vi "wait autonomous.vi"() -> ()   [LabVIEW 2010, in "Rampage.lvrbt"]
uses:
  Rampage.lvrbt
  <vilib>/NXT/Subs/MotorOutput.ctl
  <vilib>/NXT/NXTIO Xnodes/AddressXNode/NXTIOAddress.xnode
  <vilib>/NXT/Subs/MotorXNode.DC Motor Type.ctl
  <vilib>/NXT/Subs/MotorXNode.2DCMotor.ctl
  <vilib>/NXT/HiTechnic/HiTechnic Controls/HiTechnic Port.ctl
  <vilib>/NXT/Block Support/NXT_InputPort.ctl
  <vilib>/NXT/NXTIO Xnodes/NXTIOXNode/NXTIO.xnode
  <vilib>/NXT/Subs/LVHSConnector.ctl
  <vilib>/NXT/Dual Mode Library/Waits/Wait_Num(msec).vi
  <vilib>/NXT/Dual Mode Library/prims/inRangeAndCoerce/inRangeAndCoerce_int.vi
  <vilib>/NXT/Dual Mode Library/Motors/MotorOn.vi
  <vilib>/NXT/Dual Mode Library/Waits/Wait_Num.vi
  <vilib>/NXT/NXTIO Xnodes/NXTIONodeSubVIs/TETRIX IO Move DC Motors.vi
  <vilib>/NXT/NXTIO Xnodes/NXTIONodeSubVIs/TETRIX IO Stop DC Motors.vi
  <vilib>/NXT/Dual Mode Library/Sensors/Sonar_cm.vi
panel:
  out "Enabled":bool
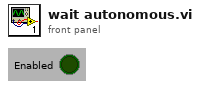
[diagram p1: front panel]
types:
  T1 = typedef "LVHSConnector.ctl" = cluster{"Hardware":string, "Flattened String":string}
  T2 = typedef "MotorOutput.ctl" = u8
  T3 = typedef "MotorXNode.DC Motor Type.ctl" = enum16{"DC Motor"}
  T4 = cluster{"DC Motor":T3, "Address":i16, "Address":i16}
  T5 = typedef "HiTechnic Port.ctl" = cluster{"Port":T6, "MUX Port":u8}
  T6 = typedef "NXT_InputPort.ctl" = u8
  T7 = cluster{"Direction (0-9)":i16, "Signal Strength (Array)":u8[]}
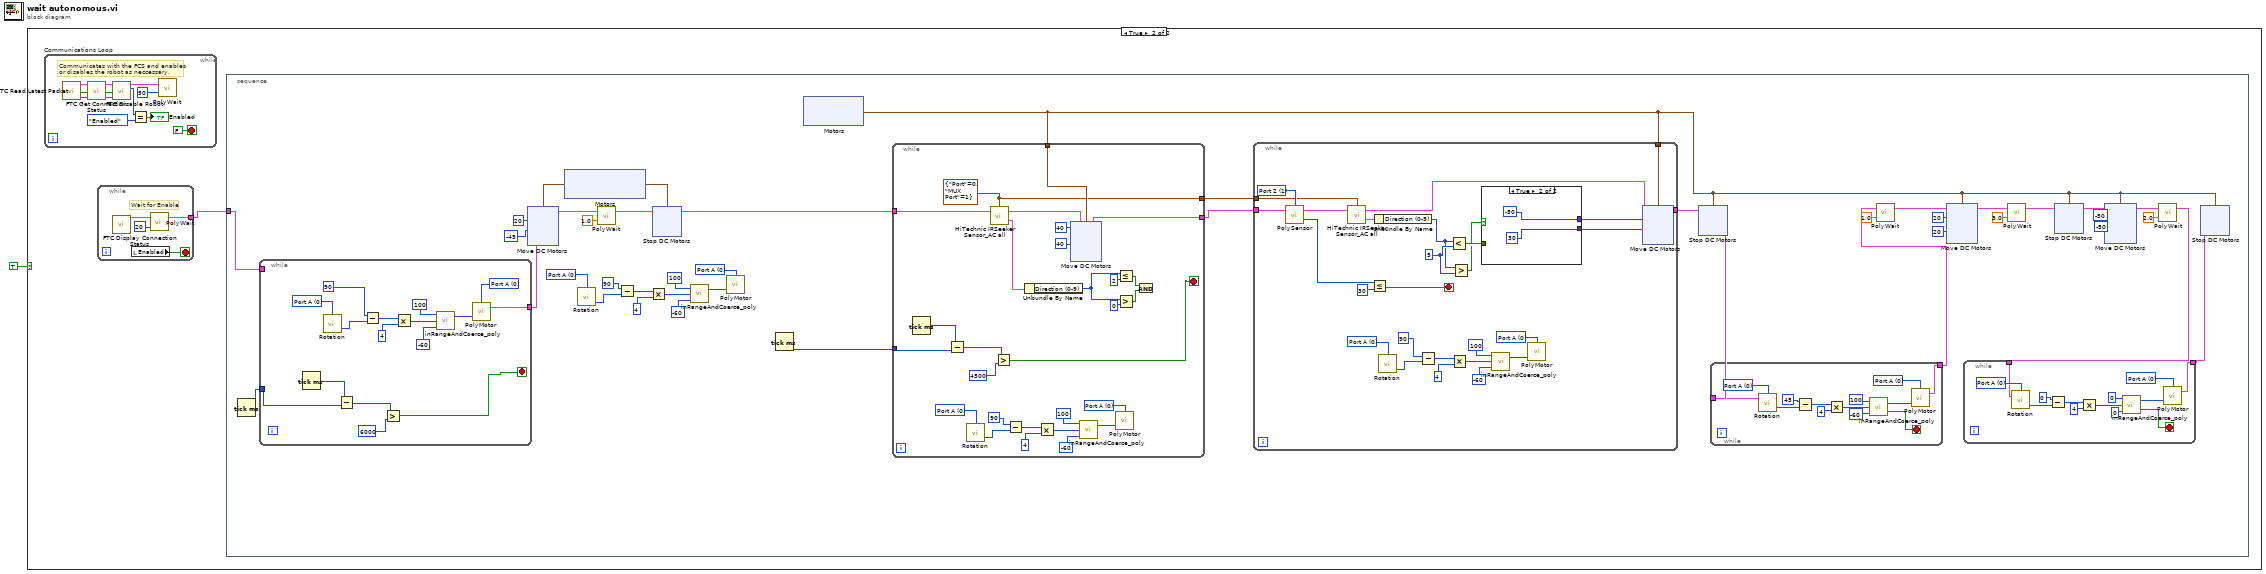
[diagram p0: block diagram]
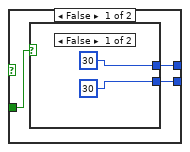
[diagram p3: hidden frame]
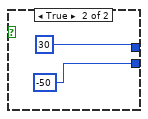
[diagram p4: hidden frame]
diagram:
  n1 = case shown="True" TRUE {
    frame False {
    }
    frame True {
      n2 = while "Communications Loop" {
        stop <- FALSE stop-if-true
        # "Communicates with the FCS and enables \nor disables the robot as neccessary."
        n3 = call <vilib>:"FTC Read Latest Packet.vi"() -> ("Packet Received?"=w243:bool, "Stopped?"=w242:bool, "NXT"=w245:T1)  [unwired: 6 in, 3 out]
        n4 = call <vilib>:"FTC Get Connection Status.vi"("Packet Received?"=w243, "Stopped?"=w242, "NXT"=w245) -> ("Online?"=w234:bool, "Stopped?"=w235:bool, "NXT"=w244:T1)  [unwired: 5 in]
        n5 = call <vilib>:"FTC Disable Robot.vi"("Online?"=w234, "Stopped?"=w235, "NXT"=w244) -> ("Enabled?"=w238:enum16{"Disabled", "Enabled"}, "NXT"=w240:T1)  [unwired: 3 in]
        n6 = Equal?(x=w238, y=enum16{"Disabled", "Enabled"}."Enabled") -> (x = y?=→"Enabled":bool)
        n7 = call-poly <vilib>:"PolyWait.vi"("Time (100 msec)"=u32 50 ("Time (msec)"), "NXT"=w240) -> ()  [unwired: 2 in, 1 out]
      }
      n8 = while {
        tunnel: [w231] -> w2
        stop <- w232 stop-if-true
        # "Wait for Enable"
        n9 = call <vilib>:"FTC Display Connection Status.vi"() -> ("NXT"=w230:T1)  [unwired: 11 in]
        n10 = local read "Enabled"() -> (w232:bool)
        n11 = call-poly <vilib>:"PolyWait.vi"("Time (100 msec)"=u32 20 ("Time (msec)"), "NXT"=w230) -> ("NXT"=w231:T1)  [unwired: 2 in]
      }
      n12 = stacked-sequence {
        tunnel: w2 -> [w8]
        frame #0 {
          w35 = T2 0 items=["Port A"=0, "Port B"=1, "Port C"=2, "Ports A & B"=4, "Ports A & C"=5, "Ports B & C"=6, "All Ports"=3] ("Output Port (All Ports)")
          w33 = u8 0 items=["Port A", "Port B", "Port C"] ("Port (Port A)")
          n13 = Tick Count (ms)() -> (millisecond timer value=w9:u32)
          n14 = while {
            tunnel: w9 -> [w72]
            tunnel: w8 -> [_]
            tunnel: [w70] -> w7
            stop <- w71 stop-if-true
            w78 = T2 0 items=["Port A"=0, "Port B"=1, "Port C"=2, "Ports A & B"=4, "Ports A & C"=5, "Ports B & C"=6, "All Ports"=3] ("Output Port (All Ports)")
            w80 = u8 0 items=["Port A", "Port B", "Port C"] ("Port (Port A)")
            n15 = Tick Count (ms)() -> (millisecond timer value=w75:u32)
            n16 = call <vilib>:"Rotation.vi"("Port (Port A)"=w80) -> ("Angle of Rotation"=w77:i32)  [unwired: 2 in, 1 out]
            n17 = Subtract(x=w75, y=w72) -> (x-y=w73:u32)
            n18 = Subtract(x=90 ("Claw\nPosition"), y=w77) -> (x-y=w79:i32)
            n19 = Greater?(x=w73, y=u32 6000) -> (0:w71:bool)
            n20 = Multiply(x=w79, y=4) -> (x*y=w81:i32)
            n21 = call-poly <vilib>:"inRangeAndCoerce_poly.vi"("lower limit"=-60, "x"=w81, "upper limit"=100) -> ("coerced(x)"=w84:i32)  [unwired: 1 out]
            n22 = call-poly <vilib>:"PolyMotor.vi"("Power (75)"=w84, "Output Port (All Ports)"=w78) -> ("NXT"=w70:T1)  [unwired: 2 in]
          }
          n23 = xnode "Motors"() -> ("DC Motor"=w43:T4)
          n24 = xnode "Move DC Motors"("Power/Speed 1"=i8 20, "Motors"=w43, "NXT"=w7, "Power/Speed 2"=i8 -45) -> ("NXT"=w41:T1)
          n25 = call <vilib>:"Rotation.vi"("Port (Port A)"=w33) -> ("Angle of Rotation"=w36:i32)  [unwired: 2 in, 1 out]
          n26 = call-poly <vilib>:"PolyWait.vi"("Time (1 sec)"=sgl 1.0, "NXT"=w41) -> ("NXT"=w38:T1)  [unwired: 2 in]
          n27 = Subtract(x=90 ("Claw\nPosition"), y=w36) -> (x-y=w34:i32)
          n28 = Multiply(x=w34, y=4) -> (x*y=w32:i32)
          n29 = xnode "Stop DC Motors"("Motors"=w43, "NXT"=w38) -> ("NXT"=w26:T1)
          n30 = call-poly <vilib>:"inRangeAndCoerce_poly.vi"("lower limit"=-60, "x"=w32, "upper limit"=100) -> ("coerced(x)"=w29:i32)  [unwired: 1 out]
          n31 = call-poly <vilib>:"PolyMotor.vi"("Power (75)"=w29, "Output Port (All Ports)"=w35) -> ()  [unwired: 2 in, 1 out]
          n32 = Tick Count (ms)() -> (millisecond timer value=w11:u32)
          n33 = xnode "Motors"() -> ("DC Motor"=w27:T4)
          n34 = while {
            tunnel: [w218] -> w10
            tunnel: w27 -> [w215]
            tunnel: [w202] -> w12
            tunnel: w26 -> [w192]
            tunnel: w11 -> [w196]
            stop <- w194 stop-if-true
            w207 = T2 0 items=["Port A"=0, "Port B"=1, "Port C"=2, "Ports A & B"=4, "Ports A & C"=5, "Ports B & C"=6, "All Ports"=3] ("Output Port (All Ports)")
            w209 = u8 0 items=["Port A", "Port B", "Port C"] ("Port (Port A)")
            w202 = T5 {"Port"=0, "MUX Port"=1} ("Port/MUX")
            n35 = Tick Count (ms)() -> (millisecond timer value=w197:u32)
            n36 = Subtract(x=w197, y=w196) -> (x-y=w193:u32)
            n37 = call <vilib>:"Rotation.vi"("Port (Port A)"=w209) -> ("Angle of Rotation"=w206:i32)  [unwired: 2 in, 1 out]
            n38 = call <vilib>:"HiTechnic IRSeeker Sensor_AC all.vi"("NXT"=w192, "Port/MUX"=w202) -> ("All Info"=w203:T7, "NXT"=w219:T1)  [unwired: 1 in]
            n39 = Greater?(x=w193, y=u32 4500) -> (0:w194:bool)
            n40 = Subtract(x=90 ("Claw\nPosition"), y=w206) -> (x-y=w208:i32)
            n41 = Unbundle By Name(w203) -> ("Direction (0-9)"=w200:i16)
            n42 = Multiply(x=w208, y=4) -> (x*y=w210:i32)
            n43 = xnode "Move DC Motors"("Power/Speed 2"=i8 40, "Power/Speed 1"=i8 40, "Motors"=w215, "NXT"=w219) -> ("NXT"=w218:T1)
            n44 = call-poly <vilib>:"inRangeAndCoerce_poly.vi"("lower limit"=-60, "x"=w210, "upper limit"=100) -> ("coerced(x)"=w213:i32)  [unwired: 1 out]
            n45 = call-poly <vilib>:"PolyMotor.vi"("Power (75)"=w213, "Output Port (All Ports)"=w207) -> ()  [unwired: 2 in, 1 out]
            n46 = Less Or Equal?(x=w200, y=i16 2) -> (x <= y?=w199:bool)
            n47 = Greater?(x=w200, y=i16 0) -> (0:w198:bool)
            n48 = And(x=w199, y=w198) -> ()  [unwired: 1 out]
          }
          n49 = while {
            tunnel: [w170] -> w15
            tunnel: w27 -> [w169]
            tunnel: w10 -> [w147]
            tunnel: w12 -> [w145]
            stop <- w146 stop-if-true
            w150 = T2 0 items=["Port A"=0, "Port B"=1, "Port C"=2, "Ports A & B"=4, "Ports A & C"=5, "Ports B & C"=6, "All Ports"=3] ("Output Port (All Ports)")
            w152 = u8 0 items=["Port A", "Port B", "Port C"] ("Port (Port A)")
            w161 = i16 5 ("y")
            w167 = T6 1 items=["Port 1", "Port 2", "Port 3", "Port 4"] ("Port (Port 4)")
            n50 = call-poly <vilib>:"PolySensor.vi"("NXT"=w147, "Port (Port 4)"=w167) -> ("Distance (cm)"=w168:i16, "NXT"=w166:T1)  [unwired: 1 in]
            n51 = call <vilib>:"HiTechnic IRSeeker Sensor_AC all.vi"("NXT"=w166, "Port/MUX"=w145) -> ("All Info"=w165:T7, "NXT"=w164:T1)  [unwired: 1 in]
            n52 = Less Or Equal?(x=w168, y=i16 30) -> (x <= y?=w146:bool)
            n53 = Unbundle By Name(w165) -> ("Direction (0-9)"=w160:i16)
            n54 = call <vilib>:"Rotation.vi"("Port (Port A)"=w152) -> ("Angle of Rotation"=w149:i32)  [unwired: 2 in, 1 out]
            n55 = Subtract(x=90 ("Claw\nPosition"), y=w149) -> (x-y=w151:i32)
            n56 = Less?(x=w160, y=w161) -> (x < y?=w159:bool)
            n57 = Multiply(x=w151, y=4) -> (x*y=w153:i32)
            n58 = Greater?(x=w160, y=w161) -> (0:w158:bool)
            n59 = case shown="True" w158 {
              tunnel: [w174 i8 -50 ("Power/Speed 2")] -> w163
              tunnel: [w173 i8 30 ("Power/Speed 1")] -> w162
              tunnel: w159 -> [w172 _]
              frame False {
                n60 = case shown="False" w172 {
                  tunnel: [i8 30 ("Power/Speed 1") i8 30 ("Power/Speed 2")] -> w174
                  tunnel: [i8 30 ("Power/Speed 2") i8 -50 ("Power/Speed 1")] -> w173
                  frame False {
                  }
                  frame True {
                  }
                }
              }
              frame True {
              }
            }
            n61 = call-poly <vilib>:"inRangeAndCoerce_poly.vi"("lower limit"=-60, "x"=w153, "upper limit"=100) -> ("coerced(x)"=w156:i32)  [unwired: 1 out]
            n62 = call-poly <vilib>:"PolyMotor.vi"("Power (75)"=w156, "Output Port (All Ports)"=w150) -> ()  [unwired: 2 in, 1 out]
            n63 = xnode "Move DC Motors"("Power/Speed 2"=w162, "Power/Speed 1"=w163, "Motors"=w169, "NXT"=w164) -> ("NXT"=w170:T1)
          }
          n64 = xnode "Stop DC Motors"("Motors"=w27, "NXT"=w15) -> ("NXT"=w6:T1)
          n65 = while {
            tunnel: w6 -> [w59]
            tunnel: [w58] -> w5
            stop <- w57 stop-if-true
            w62 = T2 0 items=["Port A"=0, "Port B"=1, "Port C"=2, "Ports A & B"=4, "Ports A & C"=5, "Ports B & C"=6, "All Ports"=3] ("Output Port (All Ports)")
            w64 = u8 0 items=["Port A", "Port B", "Port C"] ("Port (Port A)")
            n66 = call <vilib>:"Rotation.vi"("NXT"=w59, "Port (Port A)"=w64) -> ("Angle of Rotation"=w61:i32)  [unwired: 1 in, 1 out]
            n67 = Subtract(x=45 ("Claw\nPosition"), y=w61) -> (x-y=w63:i32)
            n68 = Multiply(x=w63, y=4) -> (x*y=w65:i32)
            n69 = call-poly <vilib>:"inRangeAndCoerce_poly.vi"("lower limit"=-60, "x"=w65, "upper limit"=100) -> ("In Range?"=w57:bool, "coerced(x)"=w68:i32)
            n70 = call-poly <vilib>:"PolyMotor.vi"("Power (75)"=w68, "Output Port (All Ports)"=w62) -> ("NXT"=w58:T1)  [unwired: 2 in]
          }
          n71 = call-poly <vilib>:"PolyWait.vi"("Time (1 sec)"=sgl 1.0, "NXT"=w5) -> ("NXT"=w25:T1)  [unwired: 2 in]
          n72 = xnode "Move DC Motors"("Power/Speed 2"=i8 20, "Power/Speed 1"=i8 20, "Motors"=w27, "NXT"=w25) -> ("NXT"=w18:T1)
          n73 = call-poly <vilib>:"PolyWait.vi"("Time (1 sec)"=sgl 3.0, "NXT"=w18) -> ("NXT"=w20:T1)  [unwired: 2 in]
          n74 = xnode "Stop DC Motors"("Motors"=w27, "NXT"=w20) -> ("NXT"=w21:T1)
          n75 = xnode "Move DC Motors"("Power/Speed 2"=i8 -50, "Power/Speed 1"=i8 -50, "Motors"=w27, "NXT"=w21) -> ("NXT"=w14:T1)
          n76 = call-poly <vilib>:"PolyWait.vi"("Time (1 sec)"=sgl 2.0, "NXT"=w14) -> ("NXT"=w3:T1)  [unwired: 2 in]
          n77 = while {
            tunnel: [w46] -> w4
            tunnel: w3 -> [w44]
            stop <- w45 stop-if-true
            w49 = T2 0 items=["Port A"=0, "Port B"=1, "Port C"=2, "Ports A & B"=4, "Ports A & C"=5, "Ports B & C"=6, "All Ports"=3] ("Output Port (All Ports)")
            w51 = u8 0 items=["Port A", "Port B", "Port C"] ("Port (Port A)")
            n78 = call <vilib>:"Rotation.vi"("NXT"=w44, "Port (Port A)"=w51) -> ("Angle of Rotation"=w48:i32)  [unwired: 1 in, 1 out]
            n79 = Subtract(x=0 ("Claw\nPosition"), y=w48) -> (x-y=w50:i32)
            n80 = Multiply(x=w50, y=4) -> (x*y=w52:i32)
            n81 = call-poly <vilib>:"inRangeAndCoerce_poly.vi"("lower limit"=0, "x"=w52, "upper limit"=0) -> ("In Range?"=w45:bool, "coerced(x)"=w55:i32)
            n82 = call-poly <vilib>:"PolyMotor.vi"("Power (75)"=w55, "Output Port (All Ports)"=w49) -> ("NXT"=w46:T1)  [unwired: 2 in]
          }
          n83 = xnode "Stop DC Motors"("Motors"=w27, "NXT"=w4) -> ()  [unwired: 1 out]
        }
      }
    }
  }
